vi "CRYFlatten Auto Save.vi"(11 "Auto Save":T1 {"Selector" items=["Space", "Underscores", "None"]}) -> (3 "Auto Save flattened":string)   [LabVIEW 2013]
uses:
  Typedef Control/CRYAuto Save Cluster.ctl
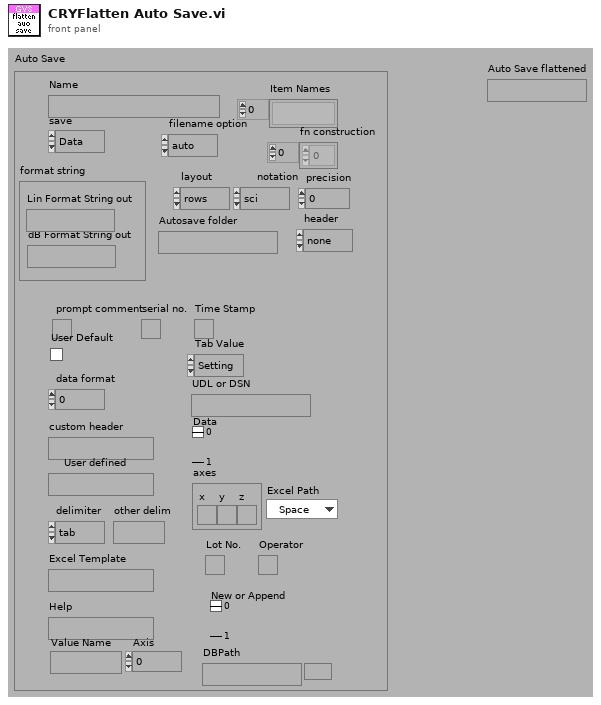
[diagram p1: front panel]
types:
  T1 = typedef "CRYAuto Save Cluster.ctl" = cluster{"Name":string, "save":enum16{"Data", "Results", "Waveforms"}, "Item Names":string[], "Autosave folder":path, "data format":u16, "filename option":enum16{"auto", "prompt"}, "fn construction":i32[], "layout":enum16{"rows", "columns"}, "notation":enum16{"sci", "float"}, "precision":i32, "prompt comment":bool, "header":enum16{"none", "standard", "custom"}, "custom header":string, "serial no.":bool, "User defined":string, "delimiter":enum16{"tab", "comma", "space", "other"}, "other delim":string, "axes":cluster{"x":bool, "y":bool, "z":bool}, "Time Stamp":bool, "Lot No.":bool, "Operator":bool, "Excel Template":string, "New or Append":u16, "Data":u16, "Help":string, "Tab Value":enum32{"Setting", "Help"}, "UDL or DSN":path, "User Default":bool, "Selector":i32, "Axis":u16, "Value Name":string, "format string":cluster{"dB Format String out":string, "Lin Format String out":string}, "DBPath":path}
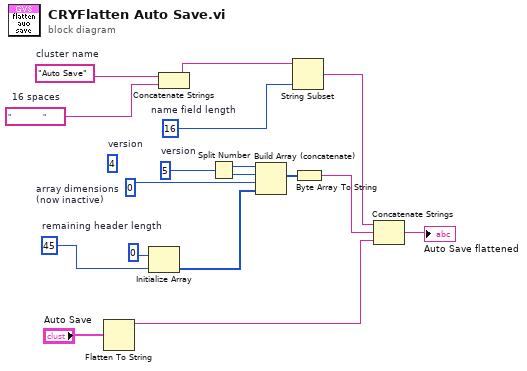
[diagram p0: block diagram]
diagram:
  (unwired) u16 4  # version
  w4 = u8 0  # array dimensions (now inactive)
  w1 = 16  # name field length
  w7 = "                "  # 16 spaces
  w8 = "Auto Save"  # cluster name
  w13 = 45  # remaining header length
  w17 = u16 5  # version
  n1 = Flatten To String(anything="Auto Save") -> (data string=w3:string)  [unwired: 1 in, 4 out]
  n2 = Initialize Array(u8 0, w13) -> (w9:u8[])
  n3 = Concatenate Strings(w8, w7) -> (w6:string)
  n4 = Split Number(x=w17) -> (hi(x)=w16:u8, lo(x)=w15:u8)
  n5 = Build Array (concatenate)(w16, w15, w4, w9) -> (w12:u8[])
  n6 = String Subset(string=w6, length (rest)=w1) -> (substring=w5:string)  [unwired: 1 out]
  n7 = Byte Array To String(unsigned byte array=w12) -> (string=w10:string)
  n8 = Concatenate Strings(w5, w10, w3) -> (→"Auto Save flattened":string)
